vi "Set Voltage and Current.vi"(0 "Yokogawa WT500 in":refnum<class "Yokogawa WT500.lvclass">, 5 "Card #":dbl, 7 "Voltage enum number":u16, 9 "Current enum number":u16, 11 "error in (no error)":errorcluster) -> (4 "Yokogawa WT500 out":refnum<class "Yokogawa WT500.lvclass">, 15 "error out":errorcluster)   [LabVIEW 2013, in "Universal Power Meter.lvlib" / "Yokogawa WT500.lvlib" / "Yokogawa WT500.lvclass"]
uses:
  Yokogawa WT500.lvclass
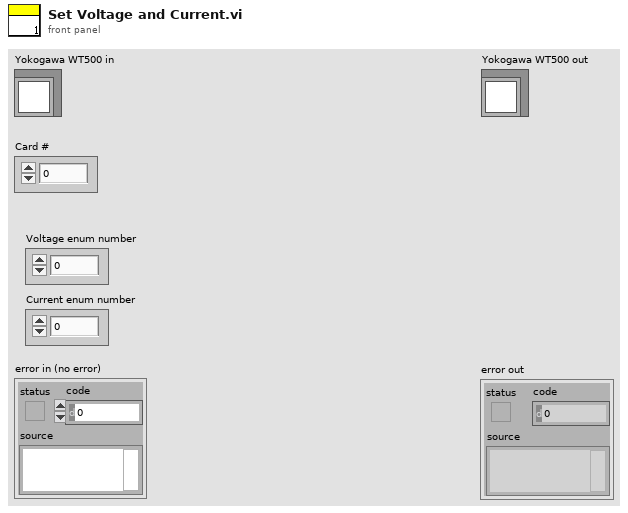
[diagram p1: front panel]
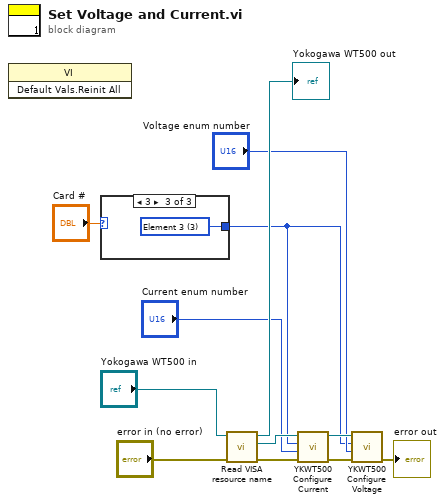
[diagram p0: block diagram]
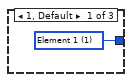
[diagram p2: hidden frame]
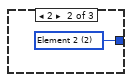
[diagram p3: hidden frame]
diagram:
  n1 = invoke class="VI" method="Default Vals.Reinit All"() -> ()  [unwired: 3 in, 3 out]
  n2 = case shown="3" "Card #" {
    tunnel: [w13 w14 w15] -> w1
    frame 1, Default {
      w13 = u16 1 items=["All", "Element 1", "Element 2", "Element 3", "Sigma"] ("Element (0: All)")
    }
    frame 2 {
      w14 = u16 2 items=["All", "Element 1", "Element 2", "Element 3", "Sigma"] ("Element (0: All)")
    }
    frame 3 {
      w15 = u16 3 items=["All", "Element 1", "Element 2", "Element 3", "Sigma"] ("Element (0: All)")
    }
  }
  n3 = call-dynamic "Read VISA resource name.vi"("error in (no error)"="error in (no error)", "Generic Instrument in"="Yokogawa WT500 in") -> ("error out"=w6:errorcluster, "VISA resource name"=w8:refnum<visa-resource-name>, "Generic Instrument out"=→"Yokogawa WT500 out":refnum<class "Yokogawa WT500.lvclass">)  [unwired: 7 in]
  n4 = call <instrlib>:"YKWT500 Configure Current.vi"("error in (no error)"=w6, "Current Range (7: 40A)"="Current enum number", "Element (0: All)"=w1, "VISA resource name"=w8) -> ("error out"=w10:errorcluster, "VISA resource name out"=w9:refnum<visa-resource-name>)  [unwired: 6 in]
  n5 = call <instrlib>:"YKWT500 Configure Voltage.vi"("error in (no error)"=w10, "Voltage Range (8: 1000V)"="Voltage enum number", "Element (0: All)"=w1, "VISA resource name"=w9) -> ("error out"=→"error out":errorcluster)  [unwired: 6 in, 1 out]
